vi "Run Tx - Untimed.vi"(7 "Process in":refnum<class "Process.lvclass">, 8 "error in (no error)":errorcluster, 11 "Tx Loop Data in":T1) -> (3 "Tx Loop Data out":T1)   [LabVIEW 2016, in "UDP-Custom-Device Engine.lvlib"]
uses:
  UDP-Custom-Device Engine.lvlib
  <vilib>/NI/NIVS Inline Async API/_VS Inline Async API/Process/Process.lvclass
  Types/Engine - Tx Loop Data.ctl
  <vilib>/NI Veristand/VeriStand Data/Byte Buffer/Byte Buffer.lvclass
  Types/Engine - General Resources.ctl
  <vilib>/NI Veristand/VeriStand Data/Typedefs/Typedefs.Data Types.ctl
  Shared/Types/Shared - Duplex Settings.ctl
  Shared/Types/Shared - Header Details.ctl
  Types/Engine - Data Conversion Config.ctl
  <vilib>/NI Veristand/VeriStand Data/Byte Buffer/Byte Buffer.Mapping.ctl
  Types/Engine - Tx Runtime Resources.ctl
  Shared/Types/Shared - Transmit Flag Options.ctl
  Types/Engine - Execution Config.ctl
  Shared/Types/Shared - Thread Management.ctl
  Types/Engine - Tx Echo Resources.ctl
  Shared/Types/Shared - Transmit Echo Options.ctl
  Types/Engine - Tx Channel Refs.ctl
  <vilib>/NI/NIVS Inline Async API/_Data Access Engine/Data Access Engine/Types/Read.DVR.ctl
  <vilib>/NI/NIVS Inline Async API/_Data Access Engine/Access Type Classes/Read/Read.lvclass
  <vilib>/NI/NIVS Inline Async API/_Data Access Engine/Data Access Engine/Types/Write.DVR.ctl
  <vilib>/NI/NIVS Inline Async API/_Data Access Engine/Access Type Classes/Write/Write.lvclass
  Types/Engine - Debug Resources.ctl
  <vilib>/NI/NIVS Inline Async API/_Data Access Engine/Access Type Classes/Read/Read.lvclass/Read.ctl
  <vilib>/NI Veristand/VeriStand Data/Byte Buffer/Byte Buffer.lvclass/Byte Buffer.ctl
  <vilib>/NI/NIVS Inline Async API/_Data Access Engine/Access Type Classes/Write/Write.lvclass/Write.ctl
  <vilib>/NI/NIVS Inline Async API/_VS Inline Async API/Process/Process.lvclass/Process.ctl
  <vilib>/NI/NIVS Inline Async API/_Data Access Engine/Data Access Engine/Methods/Data.Processes.Execute.vi
  <vilib>/NI/NIVS Inline Async API/_Data Access Engine/Data Access Engine/Methods/Read.Data.vi
  Run Tx - Handle Transmit Option.vi
  Run Tx - Handle Port Tx Check.vi
  Tx to UDP.vi
  <vilib>/NI/NIVS Inline Async API/_Data Access Engine/Data Access Engine/Methods/Write.Data.vi
  <vilib>/NI/NIVS Inline Async API/_VS Inline Async API/Error Handling Process/SubVIs/Error.ConvertArray.vi
  <vilib>/NI/NIVS Inline Async API/_Data Access Engine/Access Type Classes/Read/Read.ProcessData.vi
  <vilib>/NI Veristand/VeriStand Data/Byte Buffer/Byte Buffer.Mapping.Write.vi
  <vilib>/NI Veristand/VeriStand Data/Pointer Operations/Pointer.Write.vi
  <vilib>/NI Veristand/VeriStand Data/Pointer Operations/Pointer.Write (DBL).vi
  <vilib>/NI Veristand/VeriStand Data/Byte Buffer/Byte Buffer.Read.vi
  <vilib>/NI Veristand/VeriStand Data/Byte Buffer/Byte Buffer.Read (String).vi
  <vilib>/NI Veristand/VeriStand Data/Byte Buffer/Byte Buffer.Get Buffer Size.vi
  <vilib>/NI/NIVS Inline Async API/_Data Access Engine/Access Type Classes/Write/Write.ProcessData.vi
  <vilib>/NI Veristand/VeriStand Data/Memory Management/Memory Management.MoveDblBlock.Write (Double).vi
  <vilib>/NI Veristand/VeriStand Data/Byte Buffer/Byte Buffer.Write.Typed Double Array.vi
  <vilib>/NI Veristand/VeriStand Data/Utilities/Utilities.Buffer.Double.vi
  <vilib>/NI Veristand/VeriStand Data/Byte Buffer/Byte Buffer.Subset.Get.vi
  <vilib>/NI Veristand/VeriStand Data/Byte Buffer/Byte Buffer.Write.vi
  <vilib>/NI Veristand/VeriStand Data/Byte Buffer/Byte Buffer.Write (1D Boolean).vi
  <vilib>/NI Veristand/VeriStand Data/Type Conversion/Type Conversion.From Double.Subset.vi
  <vilib>/NI Veristand/VeriStand Data/Type Conversion/Type Conversion.From Double.Subset (1D Boolean).vi
  <vilib>/NI Veristand/VeriStand Data/Byte Buffer/Byte Buffer.Write (1D SGL).vi
  <vilib>/NI Veristand/VeriStand Data/Type Conversion/Type Conversion.From Double.Subset (1D SGL).vi
  <vilib>/NI Veristand/VeriStand Data/Byte Buffer/Byte Buffer.Write (1D DBL).vi
  <vilib>/NI Veristand/VeriStand Data/Byte Buffer/Byte Buffer.Write (1D I8).vi
  <vilib>/NI Veristand/VeriStand Data/Type Conversion/Type Conversion.From Double.Subset (1D I8).vi
  <vilib>/NI Veristand/VeriStand Data/Byte Buffer/Byte Buffer.Write (1D I16).vi
  <vilib>/NI Veristand/VeriStand Data/Type Conversion/Type Conversion.From Double.Subset (1D I16).vi
  <vilib>/NI Veristand/VeriStand Data/Byte Buffer/Byte Buffer.Write (1D I32).vi
  <vilib>/NI Veristand/VeriStand Data/Type Conversion/Type Conversion.From Double.Subset (1D I32).vi
  <vilib>/NI Veristand/VeriStand Data/Byte Buffer/Byte Buffer.Write (1D I64).vi
  <vilib>/NI Veristand/VeriStand Data/Type Conversion/Type Conversion.From Double.Subset (1D I64).vi
  <vilib>/NI Veristand/VeriStand Data/Byte Buffer/Byte Buffer.Write (1D U8).vi
  <vilib>/NI Veristand/VeriStand Data/Type Conversion/Type Conversion.From Double.Subset (1D U8).vi
  <vilib>/NI Veristand/VeriStand Data/Byte Buffer/Byte Buffer.Write (1D U16).vi
  <vilib>/NI Veristand/VeriStand Data/Type Conversion/Type Conversion.From Double.Subset (1D U16).vi
  <vilib>/NI Veristand/VeriStand Data/Byte Buffer/Byte Buffer.Write (1D U32).vi
  <vilib>/NI Veristand/VeriStand Data/Type Conversion/Type Conversion.From Double.Subset (1D U32).vi
  <vilib>/NI Veristand/VeriStand Data/Byte Buffer/Byte Buffer.Write (1D U64).vi
  <vilib>/NI Veristand/VeriStand Data/Type Conversion/Type Conversion.From Double.Subset (1D U64).vi
  <vilib>/NI Veristand/VeriStand Data/Memory Management/Memory Management.MoveByteBlock.Write (String).vi
  <vilib>/NI Veristand/VeriStand Data/Byte Buffer/Byte Buffer.Get Buffer Pointer.vi
  <vilib>/NI Veristand/VeriStand Data/Byte Buffer/Byte Buffer.Write (String).vi
  <vilib>/NI Veristand/VeriStand Data/Type Conversion/Type Conversion.From Double.vi
  <vilib>/NI Veristand/VeriStand Data/Type Conversion/Type Conversion.From Double (1D Boolean).vi
  <vilib>/NI Veristand/VeriStand Data/Type Conversion/Type Conversion.From Double (1D SGL).vi
  <vilib>/NI Veristand/VeriStand Data/Type Conversion/Type Conversion.From Double (1D I8).vi
  <vilib>/NI Veristand/VeriStand Data/Type Conversion/Type Conversion.From Double (1D I16).vi
  <vilib>/NI Veristand/VeriStand Data/Type Conversion/Type Conversion.From Double (1D I32).vi
  <vilib>/NI Veristand/VeriStand Data/Type Conversion/Type Conversion.From Double (1D I64).vi
  <vilib>/NI Veristand/VeriStand Data/Type Conversion/Type Conversion.From Double (1D U8).vi
  <vilib>/NI Veristand/VeriStand Data/Type Conversion/Type Conversion.From Double (1D U16).vi
  <vilib>/NI Veristand/VeriStand Data/Type Conversion/Type Conversion.From Double (1D U32).vi
  <vilib>/NI Veristand/VeriStand Data/Type Conversion/Type Conversion.From Double (1D U64).vi
  <vilib>/NI Veristand/VeriStand Data/Byte Buffer/Byte Buffer.Subset.Set.vi
  <vilib>/NI Veristand/VeriStand Data/Memory Management/Memory Management.MoveByteBlock.Read (String).vi
  <vilib>/NI Veristand/VeriStand Data/Memory Management/Memory Management.Handle Return.vi
  <vilib>/NI Veristand/VeriStand Data/Byte Buffer/Byte Buffer.Get Byte Order.vi
  <vilib>/NI Veristand/VeriStand Data/VeriStand Data.lvlib
  Shared/UDP-Custom-Device Shared.lvlib
  <vilib>/NI/NIVS Inline Async API/_Data Access Engine/Data Access Engine/Data Access Engine.lvclass
panel:
  out "length":i32
  out "Tx Packet":string
  # "CHANNEL TRANSMIT\n- UNTIMED\n- ALL TARGETS"
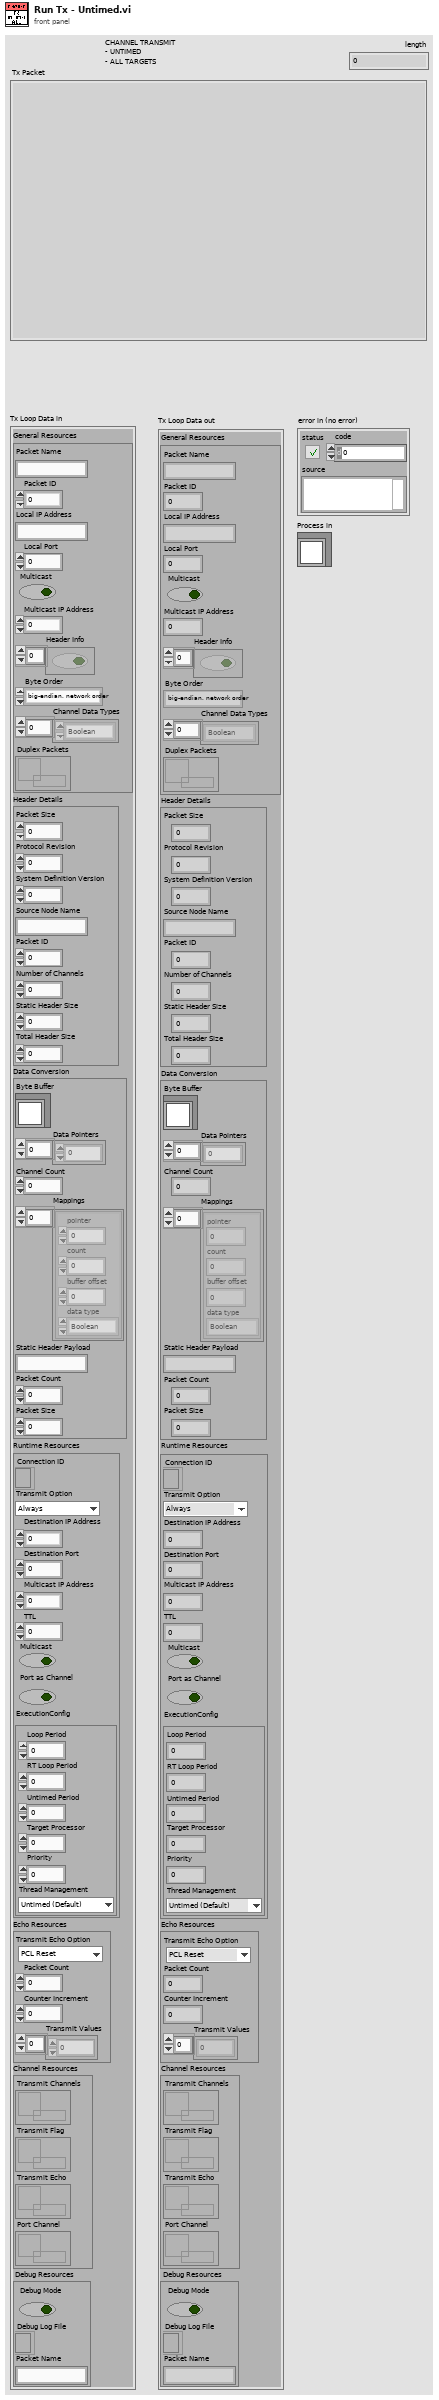
[diagram p1: front panel]
types:
  T1 = typedef "UDP-Custom-Device Engine.lvlib/Engine - Tx Loop Data.ctl" = cluster{"General Resources":T2, "Header Details":T4, "Data Conversion":T5, "Runtime Resources":T7, "Echo Resources":T11, "Channel Resources":T13, "Debug Resources":T16}
  T2 = typedef "UDP-Custom-Device Engine.lvlib/Engine - General Resources.ctl" = cluster{"Packet Name":string, "Packet ID":i32, "Local IP Address":string, "Local Port":i32, "Multicast":bool, "Multicast IP Address":u32, "Header Info":bool[], "Byte Order":enum16{"big-endian, network order", "native, host order", "little-endian"}, "Channel Data Types":T3[], "Duplex Packets":refnum<data-value>}
  T3 = typedef "VeriStand Data.lvlib/Typedefs.Data Types.ctl" = enum16{"Boolean", "Single", "Double", "I8", "I16", "I32", "I64", "U8", "U16", "U32", "U64"}
  T4 = typedef "UDP-Custom-Device Shared.lvlib/Shared - Header Details.ctl" = cluster{"Packet Size":u16, "Protocol Revision":u8, "System Definition Version":u64, "Source Node Name":string, "Packet ID":u32, "Number of Channels":u32, "Static Header Size":u16, "Total Header Size":u16}
  T5 = typedef "UDP-Custom-Device Engine.lvlib/Engine - Data Conversion Config.ctl" = cluster{"Byte Buffer":refnum<class "Byte Buffer.lvclass">, "Data Pointers":u64[], "Channel Count":i32, "Mappings":T6[], "Static Header Payload":string, "Packet Count":dbl, "Packet Size":i32}
  T6 = typedef "VeriStand Data.lvlib/Byte Buffer.lvclass/Byte Buffer.Mapping.ctl" = cluster{"pointer":u64, "count":i64, "buffer offset":u64, "data type":T3}
  T7 = typedef "UDP-Custom-Device Engine.lvlib/Engine - Tx Runtime Resources.ctl" = cluster{"Connection ID":refnum<k16>, "Transmit Option":T8, "Destination IP Address":u32, "Destination Port":u16, "Multicast IP Address":u32, "TTL":u16, "Multicast":bool, "Port as Channel":bool, "ExecutionConfig":T9}
  T8 = typedef "UDP-Custom-Device Shared.lvlib/Shared - Transmit Flag Options.ctl" = enum16{"Always", "One-Shot", "Toggle"}
  T9 = typedef "UDP-Custom-Device Engine.lvlib/Engine - Execution Config.ctl" = cluster{"Loop Period":i64, "RT Loop Period":i64, "Untimed Period":u32, "Target Processor":i32, "Priority":i32, "Thread Management":T10}
  T10 = typedef "UDP-Custom-Device Shared.lvlib/Shared - Thread Management.ctl" = enum16{"Untimed (Default)", "Timed (High Priority)"}
  T11 = typedef "UDP-Custom-Device Engine.lvlib/Engine - Tx Echo Resources.ctl" = cluster{"Transmit Echo Option":T12, "Packet Count":dbl, "Counter Increment":dbl, "Transmit Values":dbl[]}
  T12 = typedef "UDP-Custom-Device Shared.lvlib/Shared - Transmit Echo Options.ctl" = enum16{"PCL Reset", "Counter", "Mirror"}
  T13 = typedef "UDP-Custom-Device Engine.lvlib/Engine - Tx Channel Refs.ctl" = cluster{"Transmit Channels":T14, "Transmit Flag":T14, "Transmit Echo":T15, "Port Channel":T14}
  T14 = typedef "Data Access Engine.lvlib/Data Access Engine.lvclass/Read.DVR.ctl" = refnum<data-value>
  T15 = typedef "Data Access Engine.lvlib/Data Access Engine.lvclass/Write.DVR.ctl" = refnum<data-value>
  T16 = typedef "UDP-Custom-Device Engine.lvlib/Engine - Debug Resources.ctl" = cluster{"Debug Mode":bool, "Debug Log File":refnum<file>, "Packet Name":string}
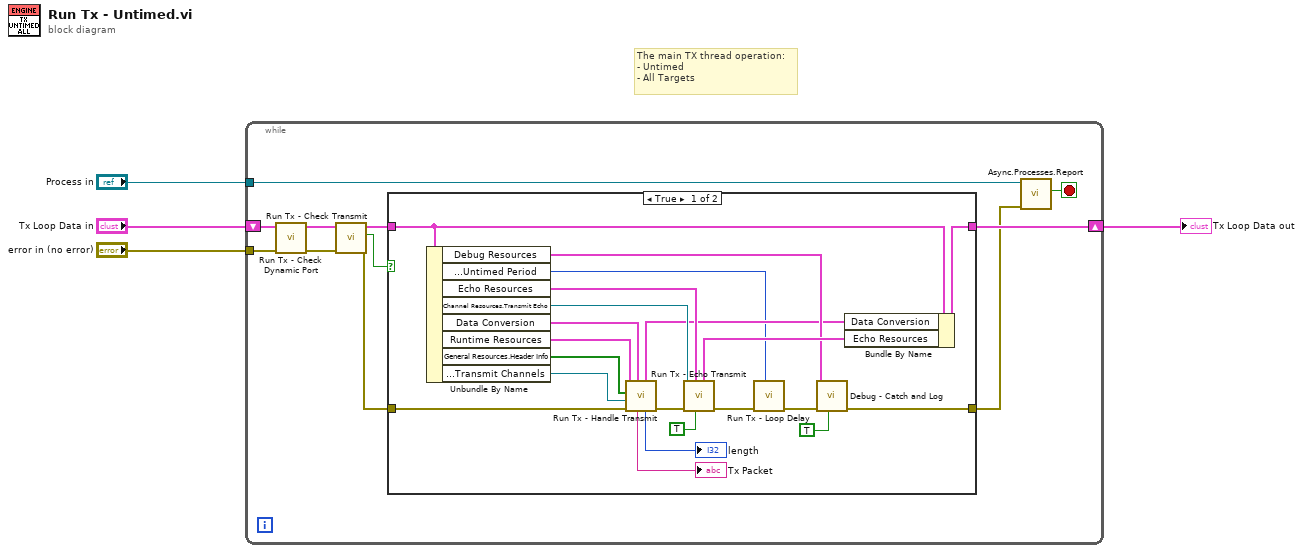
[diagram p0: block diagram]
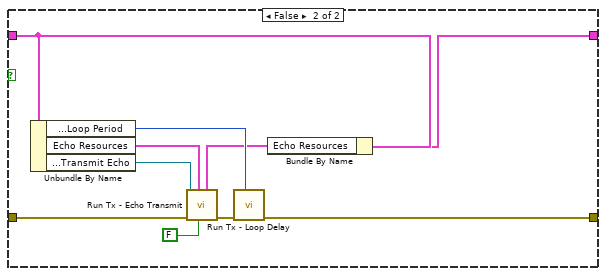
[diagram p2: hidden frame]
diagram:
  # "The main TX thread operation:\n- Untimed\n- All Targets"
  n1 = while {
    tunnel: "error in (no error)" -> [w5]
    tunnel: "Process in" -> [w15]
    shift-right: [w13] -> w1
    shift-left: "Tx Loop Data in" -> [w8]
    stop <- w14 stop-if-true
    n2 = call "Run Tx - Check Dynamic Port.vi"("error in (no error)"=w5, "Tx Loop Data in"=w8) -> ("error out"=w6:errorcluster, "Tx Loop Data out"=w7:T1)  [unwired: 8 in]
    n3 = call "Run Tx - Check Transmit.vi"("error in (no error)"=w6, "Tx Loop Data in"=w7) -> ("error out"=w11:errorcluster, "Transmit?"=w10:bool, "Tx Loop Data out"=w12:T1)  [unwired: 7 in]
    n4 = case shown="True" w10 {
      tunnel: [w30 w42] -> w9
      tunnel: [w36 w38] -> w13
      tunnel: w12 -> [w35 w39]
      tunnel: w11 -> [w22 w45]
      frame True {
        n5 = Unbundle By Name(w35) -> ("Debug Resources"=w28:T16, "Runtime Resources.ExecutionConfig.Untimed Period"=w16:u32, "Echo Resources"=w33:T11, "Channel Resources.Transmit Echo"=w34:T15, "Data Conversion"=w27:T5, "Runtime Resources"=w25:T7, "General Resources.Header Info"=w24:bool[], "Channel Resources.Transmit Channels"=w23:T14)
        n6 = call "Run Tx - Handle Transmit.vi"("Data Conversion"=w27, "error in (no error)"=w22, "Transmit Chanels"=w23, "Header Info"=w24, "Runtime Resources"=w25) -> ("error out"=w21:errorcluster, "length"=→"length":i32, "Data Conversion out"=w26:T5, "Tx Packet"=→"Tx Packet":string)  [unwired: 3 in]
        n7 = call "Run Tx - Echo Transmit.vi"("Transmitted?"=TRUE, "Echo Resources in"=w33, "error in (no error)"=w21, "Ref"=w34) -> ("error out"=w18:errorcluster, "Echo Resources out"=w32:T11)  [unwired: 6 in]
        n8 = call "Run Tx - Loop Delay.vi"("Delay (ms)"=w16, "error in (no error)"=w18) -> ("error out"=w17:errorcluster)  [unwired: 9 in]
        n9 = call "Debug - Catch and Log.vi"("Clear Error?"=TRUE, "error in (no error)"=w17, "Debug Resources"=w28) -> ("error out"=w30:errorcluster)  [unwired: 8 in]
        n10 = Bundle By Name(cluster=w35, "Data Conversion"=w26, "Echo Resources"=w32) -> (w36:T1)
      }
      frame False {
        n11 = Unbundle By Name(w39) -> ("Runtime Resources.ExecutionConfig.Loop Period"=w44:i64, "Echo Resources"=w40:T11, "Channel Resources.Transmit Echo"=w46:T15)
        n12 = call "Run Tx - Echo Transmit.vi"("Transmitted?"=FALSE, "Echo Resources in"=w40, "error in (no error)"=w45, "Ref"=w46) -> ("error out"=w43:errorcluster, "Echo Resources out"=w37:T11)  [unwired: 6 in]
        n13 = call "Run Tx - Loop Delay.vi"("Delay (ms)"=w44, "error in (no error)"=w43) -> ("error out"=w42:errorcluster)  [unwired: 9 in]
        n14 = Bundle By Name(cluster=w39, "Echo Resources"=w37) -> (w38:T1)
      }
    }
    n15 = call <vilib>:"Async.Processes.Report.vi"("Error"=w9, "Process in"=w15) -> ("Stop"=w14:bool)  [unwired: 8 in, 1 out]
  }
  "Tx Loop Data out" <- w1
